vi "诊断标定3.vi"(8 "CAN端口":u16(ring), 9 "设备索引号":u16(ring), 10 "CAN卡类型":u32(ring)=21) -> ()   [LabVIEW 2013] (continued)
                          n3577 = local write "1 7"(TRUE ("1 7")) -> ()
                        }
                        frame 2 {
                          n3578 = local write "1 8"(TRUE ("1 8")) -> ()
                        }
                        frame 3 {
                          n3579 = local write "1 9"(TRUE ("1 9")) -> ()
                        }
                        frame 5 {
                          n3580 = local write "1 10"(TRUE ("1 10")) -> ()
                        }
                        frame 4 {
                          n3581 = local write "1 12"(TRUE ("1 10")) -> ()
                        }
                      }
                      n3582 = local write "等级 2"(w5186) -> ()
                    }
                  }
                  n3583 = Array Size(array=w4905) -> (size(s)=w4904:i32)
                  n3584 = local write "命令"(w4906) -> ()
                  n3585 = Build Array(w4909) -> (w4908:u8[])
                  n3586 = while {
                    tunnel: w4906 -> [w4943]
                    tunnel: w4910 -> [w4942]
                    tunnel: w4908 -> [w4941]
                    tunnel: w4904 -> [w4937]
                    tunnel: w4901 -> [w4940]
                    tunnel: w4899 -> [w4934]
                    tunnel: [w4933] -> w4898
                    shift-right: [w4932] -> _
                    shift-left: w4907 -> [w4913]
                    shift-right: [w4923] -> _
                    shift-left: w4905 -> [w4912]
                    i -> [w4938]
                    stop <- w4933 stop-if-true
                    n3587 = local read "强制终止读写标记"() -> (w4929:bool)
                    n3588 = Array Size(array=w4913) -> (size(s)=w4931:i32)
                    n3589 = Increment(x=w4938) -> (x+1=w4939:i32)
                    n3590 = Greater Than 0?(x=w4931) -> (x > 0?=w4930:bool)
                    n3591 = Equal?(x=w4937, y=w4939) -> (x = y?=w4935:bool)
                    n3592 = Not(x=w4929) -> (.not. x?=w4928:bool)
                    n3593 = And(x=w4928, y=w4930) -> (x .and. y?=w4927:bool)
                    n3594 = Delete From Array(array=w4913, length=1 ("长度"), index=0 ("索引")) -> (deleted portion=w4919:string[], array with subset deleted=w4924:string[])
                    n3595 = Index Array(array=w4919, index=0 ("索引")) -> (element=w4917:string)
                    n3596 = Delete From Array(array=w4912, length=1 ("长度"), index=0 ("索引")) -> (deleted portion=w4915:u8[], array with subset deleted=w4920:u8[])
                    n3597 = Index Array(array=w4915, index=0 ("索引")) -> (element=w4914:u8)
                    n3598 = case shown="真" w4927 {
                      tunnel: w4943 -> [_ w4959]
                      tunnel: w4914 -> [_ w4958]
                      tunnel: w4942 -> [_ w4957]
                      tunnel: w4941 -> [_ w4956]
                      tunnel: w4917 -> [_ w4955]
                      tunnel: w4940 -> [_ w4954]
                      tunnel: w4935 -> [_ w4953]
                      tunnel: w4934 -> [_ w4952]
                      tunnel: [string[] [] w4948] -> w4932
                      tunnel: w4924 -> [_ w4951]
                      tunnel: [u8[] [] w4946] -> w4923
                      tunnel: w4920 -> [_ w4950]
                      tunnel: w4913 -> [_ w4949]
                      tunnel: w4912 -> [_ w4947]
                      frame False {
                      }
                      frame True {
                        n3599 = while {
                          tunnel: w4959 -> [w4975]
                          tunnel: w4958 -> [w4974]
                          tunnel: w4957 -> [w4973]
                          tunnel: w4956 -> [w4972]
                          tunnel: w4955 -> [w4970]
                          tunnel: w4954 -> [w4969]
                          tunnel: w4953 -> [w4968]
                          tunnel: w4952 -> [w4967]
                          tunnel: w4951 -> [w4963]
                          tunnel: w4950 -> [w4961]
                          tunnel: w4949 -> [w4964]
                          tunnel: [w4965] -> w4948
                          tunnel: w4947 -> [w4962]
                          tunnel: [w4960] -> w4946
                          i -> [w4966]
                          stop <- w4971 stop-if-true
                          n3600 = stacked-sequence {
                            seq-local: [_ _ _ _ w5122 _ _] -> [_ _ _ _ _ w5138 _]
                            tunnel: w4975 -> [_ _ _ w5114 _ _ _]
                            tunnel: w4974 -> [_ _ _ w5113 _ _ _]
                            tunnel: w4973 -> [_ _ _ w5112 _ _ _]
                            tunnel: w4972 -> [_ _ _ w5111 _ _ _]
                            tunnel: [_ _ _ _ w5123 _ _] -> w4971
                            tunnel: w4970 -> [w4977 _ _ _ _ w5137 _]
                            tunnel: w4969 -> [_ _ _ _ _ _ w5165]
                            tunnel: w4968 -> [_ _ _ _ _ _ w5163]
                            tunnel: w4967 -> [w4976 _ _ _ _ _ _]
                            tunnel: w4966 -> [_ _ _ _ _ _ _]
                            tunnel: [_ _ _ _ _ w5136 _] -> w4965
                            tunnel: w4964 -> [_ _ _ _ _ w5135 _]
                            tunnel: w4963 -> [_ _ _ _ _ w5134 _]
                            tunnel: w4962 -> [_ _ _ _ _ w5133 _]
                            tunnel: w4961 -> [_ _ _ _ _ w5132 _]
                            tunnel: [_ _ _ _ _ w5131 _] -> w4960
                            frame #0 {
                              n3601 = case shown="\"从板\"" w4976 {
                                tunnel: w4977 -> [w4978 w5069]
                                frame "主板", Default {
                                n3602 = case shown="\"电压个数\"" w4978 {
                                frame "假", Default {
                                }
                                frame "产品编号" {
                                n3603 = control-ref of="产品编号"() -> (w4980:refnum<vi>)
                                n3604 = property class="Str"(reference=w4980, "Value"="") -> ()  [unwired: 1 in, 2 out]
                                }
                                frame "电压个数" {
                                n3605 = local read "从板个数"() -> (w4981:dbl)
                                n3606 = control-ref of="项目信息"() -> (w4985:refnum<vi>)
                                n3607 = for {
                                N: w4981 -> [_]
                                tunnel: [""] -> w4984 mode=indexing
                                }
                                n3608 = call "表格数据输入-8.6.vi"("行数"=u32 0, "列数"=u32 1, "字符串数组"=w4984, "表格引用"=w4985) -> ()  [unwired: 8 in]
                                }
                                frame "通道电压数" {
                                n3609 = disable-structure shown="禁用" {
                                frame Disabled {
                                n3610 = control-ref of="项目信息"() -> (w4991:refnum<vi>)
                                n3611 = for {
                                N: 20 -> [_]
                                tunnel: [""] -> w4990 mode=indexing
                                }
                                n3612 = local read "从板个数"() -> (w4992:dbl)
                                n3613 = Increment(x=w4992) -> (x+1=w4988:dbl)
                                n3614 = call "表格数据输入-8.6.vi"("行数"=w4988, "列数"=u32 1, "字符串数组"=w4990, "表格引用"=w4991) -> ()  [unwired: 8 in]
                                }
                                frame Enabled {
                                }
                                }
                                }
                                frame "电压起始值" {
                                n3615 = disable-structure shown="禁用" {
                                frame Disabled {
                                n3616 = local read "从板个数"() -> (w4996:dbl)
                                n3617 = Increment(x=w4996) -> (x+1=w4995:dbl)
                                n3618 = control-ref of="项目信息"() -> (w5002:refnum<vi>)
                                n3619 = for {
                                N: w4995 -> [_]
                                tunnel: [""] -> w5001 mode=indexing
                                }
                                n3620 = Multiply(x=u8 1, y=w4996) -> (x*y=w4998:dbl)
                                n3621 = Add(x=w4998, y=u8 21) -> (x+y=w4994:dbl)
                                n3622 = call "表格数据输入-8.6.vi"("行数"=w4994, "列数"=u32 1, "字符串数组"=w5001, "表格引用"=w5002) -> ()  [unwired: 8 in]
                                }
                                frame Enabled {
                                }
                                }
                                }
                                frame "温度个数" {
                                n3623 = local read "从板个数"() -> (w5006:dbl)
                                n3624 = Increment(x=w5006) -> (x+1=w5005:dbl)
                                n3625 = control-ref of="项目信息"() -> (w5012:refnum<vi>)
                                n3626 = for {
                                N: w5005 -> [_]
                                tunnel: [""] -> w5011 mode=indexing
                                }
                                n3627 = Multiply(x=u8 2, y=w5006) -> (x*y=w5008:dbl)
                                n3628 = Add(x=w5008, y=u8 22) -> (x+y=w5004:dbl)
                                n3629 = call "表格数据输入-8.6.vi"("行数"=w5004, "列数"=u32 1, "字符串数组"=w5011, "表格引用"=w5012) -> ()  [unwired: 8 in]
                                }
                                frame "温度起始值" {
                                n3630 = disable-structure shown="禁用" {
                                frame Disabled {
                                n3631 = local read "从板个数"() -> (w5016:dbl)
                                n3632 = Increment(x=w5016) -> (x+1=w5015:dbl)
                                n3633 = control-ref of="项目信息"() -> (w5022:refnum<vi>)
                                n3634 = for {
                                N: w5015 -> [_]
                                tunnel: [""] -> w5021 mode=indexing
                                }
                                n3635 = Multiply(x=u8 3, y=w5016) -> (x*y=w5018:dbl)
                                n3636 = Add(x=w5018, y=u8 23) -> (x+y=w5014:dbl)
                                n3637 = call "表格数据输入-8.6.vi"("行数"=w5014, "列数"=u32 1, "字符串数组"=w5021, "表格引用"=w5022) -> ()  [unwired: 8 in]
                                }
                                frame Enabled {
                                }
                                }
                                }
                                frame "保险位置" {
                                n3638 = local read "从板个数"() -> (w5026:dbl)
                                n3639 = control-ref of="项目信息"() -> (w5032:refnum<vi>)
                                n3640 = for {
                                N: 10 -> [_]
                                tunnel: [""] -> w5031 mode=indexing
                                }
                                n3641 = Multiply(x=u8 4, y=w5026) -> (x*y=w5028:dbl)
                                n3642 = Add(x=w5028, y=u8 24) -> (x+y=w5025:dbl)
                                n3643 = call "表格数据输入-8.6.vi"("行数"=w5025, "列数"=u32 1, "字符串数组"=w5031, "表格引用"=w5032) -> ()  [unwired: 8 in]
                                }
                                frame "电池额定实际容量" {
                                w5034 = 0.0 ("值")
                                n3644 = control-ref of="电池实际容量(A)"() -> (w5035:refnum<vi>)
                                n3645 = control-ref of="电池额定容量(A)"() -> (w5036:refnum<vi>)
                                n3646 = property class="DigNum (严格)"(reference=w5035, "Value"=w5034) -> ()  [unwired: 1 in, 2 out]
                                n3647 = property class="DigNum (严格)"(reference=w5036, "Value"=w5034) -> ()  [unwired: 1 in, 2 out]
                                }
                                frame "SOC" {
                                n3648 = control-ref of="SOC(%)"() -> (w5037:refnum<vi>)
                                n3649 = property class="DigNum (严格)"(reference=w5037, "Value"=0.0 ("值")) -> ()  [unwired: 1 in, 2 out]
                                }
                                frame "配置文件版本" {
                                n3650 = control-ref of="配置文件版本"() -> (w5039:refnum<vi>)
                                n3651 = property class="Str"(reference=w5039, "Value"="" ("值")) -> ()  [unwired: 1 in, 2 out]
                                }
                                frame "参数修改记录" {
                                n3652 = control-ref of="使用者"() -> (w5042:refnum<vi>)
                                n3653 = control-ref of="系统时钟"() -> (w5043:refnum<vi>)
                                n3654 = property class="DigNum (严格)"(reference=w5042, "Value"=0.0 ("值")) -> ()  [unwired: 1 in, 2 out]
                                n3655 = property class="Str"(reference=w5043, "Value"="" ("值")) -> ()  [unwired: 1 in, 2 out]
                                }
                                frame "校正时钟" {
                                n3656 = control-ref of="系统时钟"() -> (w5045:refnum<vi>)
                                n3657 = property class="Str"(reference=w5045, "Value"="" ("值")) -> ()  [unwired: 1 in, 2 out]
                                }
                                frame "车牌号" {
                                n3658 = control-ref of="车架(牌)号"() -> (w5047:refnum<vi>)
                                n3659 = property class="Str"(reference=w5047, "Value"="" ("值")) -> ()  [unwired: 1 in, 2 out]
                                }
                                frame "SOH" {
                                n3660 = control-ref of="SOH(%)"() -> (w5050:refnum<vi>)
                                n3661 = property class="DigNum (严格)"(reference=w5050, "Value"=0.0 ("值")) -> ()  [unwired: 1 in, 2 out]
                                }
                                frame "一级故障阀值" {
                                n3662 = local write "一级故障"(T10 {"总电压过高"=0.0, "整组电压不均衡"=0.0, "SOC过高"=0.0, "单体电压过高"=0.0, "总电压过低"=0.0, "温度过高"=0.0, "温度过低"=0.0, "单组电压不均衡"=0.0, "整组温度不均衡"=0.0, "单组温度不均衡"=0.0, "单体电压过低"=0.0, "充电电流过高"=0.0, "放电电流过高"=0.0, "SOC过低"=0.0, "内阻过大"=0.0, "极柱温度过高"=0.0, "SOH过低"=0.0} ("一级故障")) -> ()
                                }
                                frame "二级故障阀值" {
                                n3663 = local write "一级故障 2"(T10 {"总电压过高"=0.0, "整组电压不均衡"=0.0, "SOC过高"=0.0, "单体电压过高"=0.0, "总电压过低"=0.0, "温度过高"=0.0, "温度过低"=0.0, "单组电压不均衡"=0.0, "整组温度不均衡"=0.0, "单组温度不均衡"=0.0, "单体电压过低"=0.0, "充电电流过高"=0.0, "放电电流过高"=0.0, "SOC过低"=0.0, "内阻过大"=0.0, "极柱温度过高"=0.0, "SOH过低"=0.0} ("一级故障")) -> ()
                                }
                                frame "三级故障阀值" {
                                n3664 = local write "一级故障 3"(T10 {"总电压过高"=0.0, "整组电压不均衡"=0.0, "SOC过高"=0.0, "单体电压过高"=0.0, "总电压过低"=0.0, "温度过高"=0.0, "温度过低"=0.0, "单组电压不均衡"=0.0, "整组温度不均衡"=0.0, "单组温度不均衡"=0.0, "单体电压过低"=0.0, "充电电流过高"=0.0, "放电电流过高"=0.0, "SOC过低"=0.0, "内阻过大"=0.0, "极柱温度过高"=0.0, "SOH过低"=0.0} ("一级故障")) -> ()
                                }
                                frame "加热控制参数" {
                                n3665 = local write "加热控制参数"(T11 {"风机开启温度"=0.0, "风机关闭温度"=0.0, "加热开启温度"=0.0, "加热关闭温度"=0.0, "风机开启温差"=0.0, "风机关闭温差"=0.0, "加热关闭温差"=0.0} ("加热控制参数")) -> ()
                                }
                                frame "充电控制参数" {
                                n3666 = local write "一级故障 5"(T12 {"最大允许单体电压"=0.0, "最大允许总电压"=0.0, "最小允许单体电压"=0.0, "最大允许充电电流"=0.0, "最小允许充电电流"=0.0, "最大允许充电温度"=0.0, "最小允许充电温度"=0.0, "电流步长"=0.0} ("一级故障 5")) -> ()
                                }
                                frame "电池信息1" {
                                w5056 = ""
                                w5057 = 0.0 ("电池串联")
                                n3667 = local read "电池信息"() -> (w5059:T13)
                                n3668 = Bundle By Name(cluster=w5059, "电池串联"=w5057, "电池并联"=w5057, "电池包额定容量"=w5057, "电池包额定能量(kWh)"=w5057, "电池包额定总电压"=w5057, "实际容量"=w5057, "电池厂家"=w5056, "电池类型"=w5056, "电池生产日期"=w5056) -> (w5058:T13)
                                n3669 = local write "电池信息"(w5058) -> ()
                                }
                                frame "电池包组号" {
                                n3670 = local read "电池信息"() -> (w5062:T13)
                                n3671 = Bundle By Name(cluster=w5062, "电池包组号"="") -> (w5061:T13)
                                n3672 = local write "电池信息"(w5061) -> ()
                                }
                                frame "充放电安时" {
                                w5063 = 0.0 ("累计充电总安时")
                                n3673 = local read "电池信息"() -> (w5065:T13)
                                n3674 = Bundle By Name(cluster=w5065, "累计充电总安时"=w5063, "累计放电总安时"=w5063) -> (w5064:T13)
                                n3675 = local write "电池信息"(w5064) -> ()
                                }
                                frame "电池充放电次数" {
                                w5066 = 0.0 ("累计充电总安时")
                                n3676 = local read "电池信息"() -> (w5068:T13)
                                n3677 = Bundle By Name(cluster=w5068, "电池充满次数"=w5066, "电池放空次数"=w5066, "电池充电次数"=w5066) -> (w5067:T13)
                                n3678 = local write "电池信息"(w5067) -> ()
                                }
                                }
                                }
                                frame "从板" {
                                n3679 = case shown="\"电压起始值\"" w5069 {
                                frame "假", Default {
                                }
                                frame "电压起始值" {
                                n3680 = control-ref of="项目信息 2"() -> (w5070:refnum<vi>)
                                n3681 = for {
                                N: 1 -> [_]
                                tunnel: [""] -> w5074 mode=indexing
                                }
                                n3682 = call "表格数据输入-8.6.vi"("行数"=u32 0, "列数"=u32 1, "字符串数组"=w5074, "表格引用"=w5070) -> ()  [unwired: 8 in]
                                }
                                frame "通道电压个数" {
                                n3683 = control-ref of="项目信息 2"() -> (w5076:refnum<vi>)
                                n3684 = for {
                                N: 5 -> [_]
                                tunnel: [""] -> w5080 mode=indexing
                                }
                                n3685 = call "表格数据输入-8.6.vi"("行数"=u32 22, "列数"=u32 1, "字符串数组"=w5080, "表格引用"=w5076) -> ()  [unwired: 8 in]
                                }
                                frame "保险位置" {
                                n3686 = control-ref of="项目信息 2"() -> (w5082:refnum<vi>)
                                n3687 = for {
                                N: 10 -> [_]
                                tunnel: [""] -> w5086 mode=indexing
                                }
                                n3688 = call "表格数据输入-8.6.vi"("行数"=u32 2, "列数"=u32 1, "字符串数组"=w5086, "表格引用"=w5082) -> ()  [unwired: 8 in]
                                }
                                frame "温度起始值" {
                                n3689 = control-ref of="项目信息 2"() -> (w5088:refnum<vi>)
                                n3690 = for {
                                N: 1 -> [_]
                                tunnel: [""] -> w5092 mode=indexing
                                }
                                n3691 = call "表格数据输入-8.6.vi"("行数"=u32 1, "列数"=u32 1, "字符串数组"=w5092, "表格引用"=w5088) -> ()  [unwired: 8 in]
                                }
                                frame "加热控制参数" {
                                n3692 = local write "加热控制参数"(T11 {"风机开启温度"=0.0, "风机关闭温度"=0.0, "加热开启温度"=0.0, "加热关闭温度"=0.0, "风机开启温差"=0.0, "风机关闭温差"=0.0, "加热关闭温差"=0.0} ("加热控制参数")) -> ()
                                }
                                frame "一级故障阀值" {
                                n3693 = local write "一级故障 6"(T15 {"电压过高"=0.0, "电压过低"=0.0, "温度过高"=0.0, "温度过低"=0.0, "电压不均衡(V)"=0.0, "温度不均衡"=0.0, "SOC过低"=0.0} ("一级故障 6")) -> ()
                                }
                                frame "二级故障阀值" {
                                n3694 = local write "一级故障 7"(T15 {"电压过高"=0.0, "电压过低"=0.0, "温度过高"=0.0, "温度过低"=0.0, "电压不均衡(V)"=0.0, "温度不均衡"=0.0, "SOC过低"=0.0} ("一级故障 7")) -> ()
                                }
                                frame "三级故障阀值" {
                                n3695 = local write "一级故障 8"(T15 {"电压过高"=0.0, "电压过低"=0.0, "温度过高"=0.0, "温度过低"=0.0, "电压不均衡(V)"=0.0, "温度不均衡"=0.0, "SOC过低"=0.0} ("一级故障 7")) -> ()
                                }
                                frame "均衡参数" {
                                n3696 = local write "均衡参数"(T17 {"充电结束电压(90%)"=0.0, "充电结束电压(91%)"=0.0, "充电结束电压(92%)"=0.0, "充电结束电压(93%)"=0.0, "充电结束电压(94%)"=0.0, "均衡计算-电压高阀值1级"=0.0, "均衡计算-电压高阀值2级"=0.0, "均衡计算-电压低阀值1级"=0.0, "均衡计算-电压低阀值2级"=0.0, "均衡计算-最低电压阀值"=0.0, "均衡停止-最低电压阀值"=0.0, "均衡计算-电压极差阀值"=0.0, "充电结束电压(95%)"=0.0, "充电结束电压(96%)"=0.0, "充电结束电压(97%)"=0.0, "充电结束电压(98%)"=0.0, "充电结束电压(99%)"=0.0, "充电结束电压(100%)"=0.0} ("均衡参数")) -> ()
                                }
                                frame "均衡阀值" {
                                w5099 = sgl 0.0 ("均衡计算-电压高阀值1级")
                                n3697 = local read "均衡参数"() -> (w5100:T17)
                                n3698 = Bundle By Name(cluster=w5100, "均衡计算-电压高阀值1级"=w5099, "均衡计算-电压高阀值2级"=w5099, "均衡计算-电压低阀值1级"=w5099, "均衡计算-电压低阀值2级"=w5099, "均衡计算-最低电压阀值"=w5099, "均衡停止-最低电压阀值"=w5099, "均衡计算-电压极差阀值"=w5099) -> (w5101:T17)
                                n3699 = local write "均衡参数"(w5101) -> ()
                                }
                                frame "充电结束电压" {
                                w5102 = sgl 0.0 ("均衡计算-电压高阀值1级")
                                n3700 = local read "均衡参数"() -> (w5103:T17)
                                n3701 = Bundle By Name(cluster=w5103, "充电结束电压(90%)"=w5102, "充电结束电压(91%)"=w5102, "充电结束电压(92%)"=w5102, "充电结束电压(93%)"=w5102, "充电结束电压(94%)"=w5102, "充电结束电压(95%)"=w5102, "充电结束电压(96%)"=w5102, "充电结束电压(97%)"=w5102, "充电结束电压(98%)"=w5102, "充电结束电压(99%)"=w5102, "充电结束电压(100%)"=w5102) -> (w5104:T17)
                                n3702 = local write "均衡参数"(w5104) -> ()
                                }
                                }
                                }
                              }
                            }
                            frame #1 {
                              w5105 = FALSE ("流控帧")
                              w5106 = TRUE ("流控帧 2")
                              n3703 = global write "EV05全局变量1.vi" "写入超时"(w5105) -> ()
                              n3704 = global write "EV05全局变量1.vi" "流控帧"(w5105) -> ()
                              n3705 = local write "写?"(w5105) -> ()
                              n3706 = local write "消除"(w5106) -> ()
                              n3707 = local write "控制1"(w5106) -> ()
                              n3708 = global write "EV05全局变量1.vi" "流控帧 2"(w5106) -> ()
                            }
                            frame #2 {
                              n3709 = Wait Until Next ms Multiple(millisecond multiple=u32 300 ("毫秒倍数")) -> ()  [unwired: 1 out]
                            }
                            frame #3 {
                              n3710 = local read "设备索引号"() -> (w5109:u16)
                              n3711 = local read "CAN卡类型"() -> (w5110:u32)
                              n3712 = local read "CAN端口"() -> (w5108:u16)
                              n3713 = local write "命令序号"(w5113) -> ()
                              n3714 = stacked-sequence {
                                tunnel: w5114 -> [_ w5121]
                                tunnel: w5113 -> [_ w5120]
                                tunnel: w5112 -> [_ w5119]
                                tunnel: w5111 -> [_ w5118]
                                tunnel: w5110 -> [_ w5117]
                                tunnel: w5109 -> [_ w5116]
                                tunnel: w5108 -> [_ w5115]
                                frame #0 {
                                }
                                frame #1 {
                                n3715 = call "多帧发送机制(EV05).vi"("can卡类型"=w5117, "设备索引号"=w5116, "CAN端口"=w5115, "命令"=w5121, "板号"=w5119, "命令序号"=w5120, "输入数据"=w5118) -> ()  [unwired: 1 in, 12 out]
                                }
                              }
                            }
                            frame #4 {
                              n3716 = while {
                                tunnel: [w5126] -> w5123
                                tunnel: [w5125] -> w5122
                                i -> [w5129]
                                stop <- w5126 stop-if-true
                                n3717 = local read "强制终止读写标记"() -> (w5124:bool)
                                n3718 = global read "EV05全局变量1.vi" "写入超时"() -> (w5125:bool)
                                n3719 = Greater Or Equal?(x=w5129, y=20) -> (x >= y?=w5127:bool)
                                n3720 = Compound Arithmetic op=OR(w5124, w5125, w5127) -> (w5126:bool)
                                n3721 = Wait Until Next ms Multiple(millisecond multiple=u32 100 ("毫秒倍数")) -> ()  [unwired: 1 out]
                              }
                            }
                            frame #5 {
                              n3722 = case shown="假" w5138 {
                                tunnel: w5137 -> [w5149 _]
                                tunnel: [w5144 w5161] -> w5136
                                tunnel: w5135 -> [w5143 _]
                                tunnel: w5134 -> [w5142 w5161]
                                tunnel: [w5141 w5160] -> w5131
                                tunnel: w5133 -> [w5140 _]
                                tunnel: w5132 -> [w5139 w5160]
                                frame False {
                                n3723 = local read "重试次数"() -> (w5148:u8)
                                n3724 = Increment(x=w5148) -> (x+1=w5147:u8)
                                n3725 = local write "重试次数"(w5147) -> ()
                                n3726 = Greater Or Equal?(x=w5147, y=u8 4) -> (x >= y?=w5146:bool)
                                n3727 = case shown="真" w5146 {
                                tunnel: w5149 -> [_ w5154]
                                tunnel: [w5151 w5153] -> w5144
                                tunnel: w5143 -> [w5151 _]
                                tunnel: w5142 -> [_ w5153]
                                tunnel: [w5150 w5152] -> w5141
                                tunnel: w5140 -> [w5150 _]
                                tunnel: w5139 -> [_ w5152]
                                frame False {
                                }
                                frame True {
                                n3728 = control-ref of="结果"() -> (w5156:refnum<vi>)
                                n3729 = Concatenate Strings(w5154, "     读取失败" ("字符串")) -> (w5158:string)
                                n3730 = Build Array(w5158) -> (w5155:string[])
                                n3731 = call "表格编辑.vi"("新元素/子数组"=w5155, "活动单元格:单元格背景色"=u32 16740749, "MCListbox引用句柄"=w5156) -> ()  [unwired: 9 out]
                                }
                                }
                                }
                                frame True {
                                }
                              }
                            }
                            frame #6 {
                              n3732 = And(x=w5163, y=w5165) -> (x .and. y?=w5164:bool)
                              n3733 = case shown="真" w5164 {
                                frame False {
                                }
                                frame True {
                                n3734 = local write "强制终止读写标记"(FALSE ("强制停止")) -> ()
                                n3735 = control-ref of="结果"() -> (w5168:refnum<vi>)
                                n3736 = Concatenate Strings("读取完成" ("字符串")) -> (w5170:string)
                                n3737 = Build Array(w5170) -> (w5167:string[])
                                n3738 = call "表格编辑.vi"("新元素/子数组"=w5167, "活动单元格:单元格背景色"=u32 21937, "MCListbox引用句柄"=w5168) -> ()  [unwired: 9 out]
                                }
                              }
                              n3739 = Wait (ms)(milliseconds to wait=u32 100 ("等待时间（毫秒）")) -> ()  [unwired: 1 out]
                            }
                          }
                        }
                      }
                    }
                    n3740 = local read "强制终止读写标记"() -> (w4936:bool)
                    n3741 = Or(x=w4936, y=w4935) -> (x .or. y?=w4933:bool)
                  }
                }
              }
              frame #2 {
                n3742 = case shown="假" w5261 {
                  tunnel: w5262 -> [w5263 _]
                  frame False {
                    n3743 = case shown="\"主板\", 默认" w5263 {
                      frame "主板", Default {
                        n3744 = global read "读配置文件全局.vi" "电池额定实际容量判定"() -> (w5277:bool)
                        n3745 = global read "读配置文件全局.vi" "电池充放电次数判定"() -> (w5266:bool)
                        n3746 = global read "读配置文件全局.vi" "加热控制参数判定"() -> (w5264:bool)
                        n3747 = global read "读配置文件全局.vi" "配置文件版本判定"() -> (w5276:bool)
                        n3748 = global read "读配置文件全局.vi" "充电控制参数判定"() -> (w5270:bool)
                        n3749 = global read "读配置文件全局.vi" "通道电压数判定"() -> (w5282:bool)
                        n3750 = global read "读配置文件全局.vi" "电压起始值判定"() -> (w5281:bool)
                        n3751 = global read "读配置文件全局.vi" "温度起始值判定"() -> (w5279:bool)
                        n3752 = global read "读配置文件全局.vi" "充放电安时判定"() -> (w5268:bool)
                        n3753 = global read "读配置文件全局.vi" "电池包组号判定"() -> (w5267:bool)
                        n3754 = global read "读配置文件全局.vi" "电池信息1判定"() -> (w5269:bool)
                        n3755 = global read "读配置文件全局.vi" "从板个数判定"() -> (w5285:bool)
                        n3756 = global read "读配置文件全局.vi" "产品编号判定"() -> (w5284:bool)
                        n3757 = global read "读配置文件全局.vi" "电压个数判定"() -> (w5283:bool)
                        n3758 = global read "读配置文件全局.vi" "温度个数判定"() -> (w5280:bool)
                        n3759 = global read "读配置文件全局.vi" "保险位置判定"() -> (w5278:bool)
                        n3760 = global read "读配置文件全局.vi" "一级故障判定"() -> (w5273:bool)
                        n3761 = global read "读配置文件全局.vi" "二级故障判定"() -> (w5272:bool)
                        n3762 = global read "读配置文件全局.vi" "三级故障判定"() -> (w5271:bool)
                        n3763 = global read "读配置文件全局.vi" "车牌号判定"() -> (w5275:bool)
                        n3764 = global read "读配置文件全局.vi" "SOH判定"() -> (w5274:bool)
                        n3765 = Build Array(w5285, w5284, w5283, w5282, w5281, w5280, w5279, w5278, w5277, w5276, w5275, w5274, w5273, w5272, w5271, w5270, w5269, w5268, w5267, w5266, w5264) -> (w5265:bool[])
                        n3766 = And Array Elements(Boolean array=w5265) -> (logical AND=w5286:bool)
                        n3767 = disable-structure shown="禁用" {
                          frame Disabled {
                            n3768 = global read "读配置文件全局.vi" "SOC判定"() -> ()  [unwired: 1 out]
                          }
                          frame Enabled {
                          }
                        }
                        n3769 = case shown="假" w5286 {
                          tunnel: w5265 -> [_ w5291]
                          frame True {
                            n3770 = control-ref of="结果"() -> (w5289:refnum<vi>)
                            n3771 = Build Array("全部判定成功!!!!!!!!") -> (w5290:string[])
                            n3772 = call "表格编辑.vi"("新元素/子数组"=w5290, "活动单元格:单元格背景色"=u32 6618880, "MCListbox引用句柄"=w5289) -> ()  [unwired: 9 out]
                          }
                          frame False {
                            n3773 = stacked-sequence {
                              tunnel: w5291 -> [_ w5296]
                              frame #0 {
                                n3774 = control-ref of="结果"() -> (w5294:refnum<vi>)
                                n3775 = Build Array("全部判定失败!!!!!") -> (w5295:string[])
                                n3776 = call "表格编辑.vi"("新元素/子数组"=w5295, "活动单元格:单元格背景色"=u32 16711680, "MCListbox引用句柄"=w5294) -> ()  [unwired: 9 out]
                              }
                              frame #1 {
                                n3777 = for {
                                tunnel: w5296 -> [w5298] mode=indexing
                                i -> [w5297]
                                n3778 = case shown="20" w5297 {
                                tunnel: w5298 -> [w5299 w5304 w5309 w5314 w5319 w5324 w5329 w5334 w5339 w5344 w5349 w5354 w5359 w5364 w5369 w5374 w5379 w5384 w5389 w5394 w5399 _]
                                frame 0 {
                                n3779 = case shown="假" w5299 {
                                frame False {
                                n3780 = control-ref of="结果"() -> (w5302:refnum<vi>)
                                n3781 = Build Array("从板个数判定失败!") -> (w5303:string[])
                                n3782 = call "表格编辑.vi"("新元素/子数组"=w5303, "活动单元格:单元格背景色"=u32 16711680, "MCListbox引用句柄"=w5302) -> ()  [unwired: 9 out]
                                }
                                frame True {
                                }
                                }
                                }
                                frame 1 {
                                n3783 = case shown="假" w5304 {
                                frame False {
                                n3784 = control-ref of="结果"() -> (w5307:refnum<vi>)
                                n3785 = Build Array("产品编号判定失败!") -> (w5308:string[])
                                n3786 = call "表格编辑.vi"("新元素/子数组"=w5308, "活动单元格:单元格背景色"=u32 16711680, "MCListbox引用句柄"=w5307) -> ()  [unwired: 9 out]
                                }
                                frame True {
                                }
                                }
                                }
                                frame 2 {
                                n3787 = case shown="假" w5309 {
                                frame False {
                                n3788 = control-ref of="结果"() -> (w5312:refnum<vi>)
                                n3789 = Build Array("电压个数判定失败!") -> (w5313:string[])
                                n3790 = call "表格编辑.vi"("新元素/子数组"=w5313, "活动单元格:单元格背景色"=u32 16711680, "MCListbox引用句柄"=w5312) -> ()  [unwired: 9 out]
                                }
                                frame True {
                                }
                                }
                                }
                                frame 3 {
                                n3791 = case shown="假" w5314 {
                                frame False {
                                n3792 = control-ref of="结果"() -> (w5317:refnum<vi>)
                                n3793 = Build Array("通道电压数判定失败!") -> (w5318:string[])
                                n3794 = call "表格编辑.vi"("新元素/子数组"=w5318, "活动单元格:单元格背景色"=u32 16711680, "MCListbox引用句柄"=w5317) -> ()  [unwired: 9 out]
                                }
                                frame True {
                                }
                                }
                                }
                                frame 4 {
                                n3795 = case shown="假" w5319 {
                                frame False {
                                n3796 = control-ref of="结果"() -> (w5322:refnum<vi>)
                                n3797 = Build Array("电压起始值判定失败!") -> (w5323:string[])
                                n3798 = call "表格编辑.vi"("新元素/子数组"=w5323, "活动单元格:单元格背景色"=u32 16711680, "MCListbox引用句柄"=w5322) -> ()  [unwired: 9 out]
                                }
                                frame True {
                                }
                                }
                                }
                                frame 5 {
                                n3799 = case shown="假" w5324 {
                                frame False {
                                n3800 = control-ref of="结果"() -> (w5327:refnum<vi>)
                                n3801 = Build Array("温度个数判定失败!") -> (w5328:string[])
                                n3802 = call "表格编辑.vi"("新元素/子数组"=w5328, "活动单元格:单元格背景色"=u32 16711680, "MCListbox引用句柄"=w5327) -> ()  [unwired: 9 out]
                                }
                                frame True {
                                }
                                }
                                }
                                frame 6 {
                                n3803 = case shown="假" w5329 {
                                frame False {
                                n3804 = control-ref of="结果"() -> (w5332:refnum<vi>)
                                n3805 = Build Array("温度起始值判定失败!") -> (w5333:string[])
                                n3806 = call "表格编辑.vi"("新元素/子数组"=w5333, "活动单元格:单元格背景色"=u32 16711680, "MCListbox引用句柄"=w5332) -> ()  [unwired: 9 out]
                                }
                                frame True {
                                }
                                }
                                }
                                frame 7 {
                                n3807 = case shown="假" w5334 {
                                frame False {
                                n3808 = control-ref of="结果"() -> (w5337:refnum<vi>)
                                n3809 = Build Array("保险位置判定失败!") -> (w5338:string[])
                                n3810 = call "表格编辑.vi"("新元素/子数组"=w5338, "活动单元格:单元格背景色"=u32 16711680, "MCListbox引用句柄"=w5337) -> ()  [unwired: 9 out]
                                }
                                frame True {
                                }
                                }
                                }
                                frame 8 {
                                n3811 = case shown="假" w5339 {
                                frame False {
                                n3812 = control-ref of="结果"() -> (w5342:refnum<vi>)
                                n3813 = Build Array("电池额定实际容量判定失败!") -> (w5343:string[])
                                n3814 = call "表格编辑.vi"("新元素/子数组"=w5343, "活动单元格:单元格背景色"=u32 16711680, "MCListbox引用句柄"=w5342) -> ()  [unwired: 9 out]
                                }
                                frame True {
                                }
                                }
                                }
                                frame 9 {
                                n3815 = case shown="假" w5344 {
                                frame False {
                                n3816 = control-ref of="结果"() -> (w5347:refnum<vi>)
                                n3817 = Build Array("配置文件版本判定失败!") -> (w5348:string[])
                                n3818 = call "表格编辑.vi"("新元素/子数组"=w5348, "活动单元格:单元格背景色"=u32 16711680, "MCListbox引用句柄"=w5347) -> ()  [unwired: 9 out]
                                }
                                frame True {
                                }
                                }
                                }
                                frame 10 {
                                n3819 = case shown="假" w5349 {
                                frame False {
                                n3820 = control-ref of="结果"() -> (w5352:refnum<vi>)
                                n3821 = Build Array("车牌号判定失败!") -> (w5353:string[])
                                n3822 = call "表格编辑.vi"("新元素/子数组"=w5353, "活动单元格:单元格背景色"=u32 16711680, "MCListbox引用句柄"=w5352) -> ()  [unwired: 9 out]
                                }
                                frame True {
                                }
                                }
                                }
                                frame 11 {
                                n3823 = case shown="假" w5354 {
                                frame False {
                                n3824 = control-ref of="结果"() -> (w5357:refnum<vi>)
                                n3825 = Build Array("SOH判定失败!") -> (w5358:string[])
                                n3826 = call "表格编辑.vi"("新元素/子数组"=w5358, "活动单元格:单元格背景色"=u32 16711680, "MCListbox引用句柄"=w5357) -> ()  [unwired: 9 out]
                                }
                                frame True {
                                }
                                }
                                }
                                frame 12 {
                                n3827 = case shown="假" w5359 {
                                frame False {
                                n3828 = control-ref of="结果"() -> (w5362:refnum<vi>)
                                n3829 = Build Array("一级故障阀值判定失败!") -> (w5363:string[])
                                n3830 = call "表格编辑.vi"("新元素/子数组"=w5363, "活动单元格:单元格背景色"=u32 16711680, "MCListbox引用句柄"=w5362) -> ()  [unwired: 9 out]
                                }
                                frame True {
                                }
                                }
                                }
                                frame 13 {
                                n3831 = case shown="假" w5364 {
                                frame False {
                                n3832 = control-ref of="结果"() -> (w5367:refnum<vi>)
                                n3833 = Build Array("二级故障阀值判定失败!") -> (w5368:string[])
                                n3834 = call "表格编辑.vi"("新元素/子数组"=w5368, "活动单元格:单元格背景色"=u32 16711680, "MCListbox引用句柄"=w5367) -> ()  [unwired: 9 out]
                                }
                                frame True {
                                }
                                }
                                }
                                frame 14 {
                                n3835 = case shown="假" w5369 {
                                frame False {
                                n3836 = control-ref of="结果"() -> (w5372:refnum<vi>)
                                n3837 = Build Array("三级故障阀值判定失败!") -> (w5373:string[])
                                n3838 = call "表格编辑.vi"("新元素/子数组"=w5373, "活动单元格:单元格背景色"=u32 16711680, "MCListbox引用句柄"=w5372) -> ()  [unwired: 9 out]
                                }
                                frame True {
                                }
                                }
                                }
                                frame 15 {
                                n3839 = case shown="假" w5374 {
                                frame False {
                                n3840 = control-ref of="结果"() -> (w5377:refnum<vi>)
                                n3841 = Build Array("充电控制参数判定失败!") -> (w5378:string[])
                                n3842 = call "表格编辑.vi"("新元素/子数组"=w5378, "活动单元格:单元格背景色"=u32 16711680, "MCListbox引用句柄"=w5377) -> ()  [unwired: 9 out]
                                }
                                frame True {
                                }
                                }
                                }
                                frame 16 {
                                n3843 = case shown="假" w5379 {
                                frame False {
                                n3844 = control-ref of="结果"() -> (w5382:refnum<vi>)
                                n3845 = Build Array("电池信息1判定失败!") -> (w5383:string[])
                                n3846 = call "表格编辑.vi"("新元素/子数组"=w5383, "活动单元格:单元格背景色"=u32 16711680, "MCListbox引用句柄"=w5382) -> ()  [unwired: 9 out]
                                }
                                frame True {
                                }
                                }
                                }
                                frame 17 {
                                n3847 = case shown="假" w5384 {
                                frame False {
                                n3848 = control-ref of="结果"() -> (w5387:refnum<vi>)
                                n3849 = Build Array("充放电安时判定失败!") -> (w5388:string[])
                                n3850 = call "表格编辑.vi"("新元素/子数组"=w5388, "活动单元格:单元格背景色"=u32 16711680, "MCListbox引用句柄"=w5387) -> ()  [unwired: 9 out]
                                }
                                frame True {
                                }
                                }
                                }
                                frame 18 {
                                n3851 = case shown="假" w5389 {
                                frame False {
                                n3852 = control-ref of="结果"() -> (w5392:refnum<vi>)
                                n3853 = Build Array("电池包组号判定失败!") -> (w5393:string[])
                                n3854 = call "表格编辑.vi"("新元素/子数组"=w5393, "活动单元格:单元格背景色"=u32 16711680, "MCListbox引用句柄"=w5392) -> ()  [unwired: 9 out]
                                }
                                frame True {
                                }
                                }
                                }
                                frame 19 {
                                n3855 = case shown="假" w5394 {
                                frame False {
                                n3856 = control-ref of="结果"() -> (w5397:refnum<vi>)
                                n3857 = Build Array("电池充放电次数判定失败!") -> (w5398:string[])
                                n3858 = call "表格编辑.vi"("新元素/子数组"=w5398, "活动单元格:单元格背景色"=u32 16711680, "MCListbox引用句柄"=w5397) -> ()  [unwired: 9 out]
                                }
                                frame True {
                                }
                                }
                                }
                                frame 20 {
                                n3859 = case shown="假" w5399 {
                                frame False {
                                n3860 = control-ref of="结果"() -> (w5402:refnum<vi>)
                                n3861 = Build Array("加热控制参数判定失败!") -> (w5403:string[])
                                n3862 = call "表格编辑.vi"("新元素/子数组"=w5403, "活动单元格:单元格背景色"=u32 16711680, "MCListbox引用句柄"=w5402) -> ()  [unwired: 9 out]
                                }
                                frame True {
                                }
                                }
                                }
                                frame 99, Default {
                                }
                                }
                                }
                              }
                            }
                          }
                        }
                      }
                      frame "从板" {
                        n3863 = global read "读配置文件全局2.vi" "电压起始值判定"() -> (w5412:bool)
                        n3864 = global read "读配置文件全局2.vi" "温度起始值判定"() -> (w5409:bool)
                        n3865 = global read "读配置文件全局2.vi" "加热控制参数判定"() -> (w5404:bool)
                        n3866 = global read "读配置文件全局2.vi" "通道电压判定"() -> (w5411:bool)
                        n3867 = global read "读配置文件全局2.vi" "保险位置判定"() -> (w5410:bool)
                        n3868 = global read "读配置文件全局2.vi" "一级故障判定"() -> (w5407:bool)
                        n3869 = global read "读配置文件全局2.vi" "二级故障判定"() -> (w5406:bool)
                        n3870 = global read "读配置文件全局2.vi" "三级故障判定"() -> (w5405:bool)
                        n3871 = global read "读配置文件全局2.vi" "从板号判定"() -> (w5413:bool)
                        n3872 = Build Array(w5413, w5412, w5411, w5410, w5409, w5407, w5406, w5405, w5404) -> (w5408:bool[])
                        n3873 = And Array Elements(Boolean array=w5408) -> (logical AND=w5414:bool)
                        n3874 = case shown="假" w5414 {
                          tunnel: w5408 -> [_ w5419]
                          frame True {
                            n3875 = control-ref of="结果"() -> (w5417:refnum<vi>)
                            n3876 = Build Array("读取判定成功!!!!!!!!") -> (w5418:string[])
                            n3877 = call "表格编辑.vi"("新元素/子数组"=w5418, "活动单元格:单元格背景色"=u32 6618880, "MCListbox引用句柄"=w5417) -> ()  [unwired: 9 out]
                          }
                          frame False {
                            n3878 = stacked-sequence {
                              tunnel: w5419 -> [_ w5424]
                              frame #0 {
                                n3879 = control-ref of="结果"() -> (w5422:refnum<vi>)
                                n3880 = Build Array("读取判定失败!!!!!") -> (w5423:string[])
                                n3881 = call "表格编辑.vi"("新元素/子数组"=w5423, "活动单元格:单元格背景色"=u32 16711680, "MCListbox引用句柄"=w5422) -> ()  [unwired: 9 out]
                              }
                              frame #1 {
                                n3882 = for {
                                tunnel: w5424 -> [w5425] mode=indexing
                                i -> [w5426]
                                n3883 = case shown="0" w5426 {
                                tunnel: w5425 -> [w5427 w5432 w5437 w5442 w5447 w5452 w5457 w5462 w5467 _]
                                frame 0 {
                                n3884 = case shown="假" w5427 {
                                frame False {
                                n3885 = control-ref of="结果"() -> (w5430:refnum<vi>)
                                n3886 = Build Array("从板号判定失败!") -> (w5431:string[])
                                n3887 = call "表格编辑.vi"("新元素/子数组"=w5431, "活动单元格:单元格背景色"=u32 16711680, "MCListbox引用句柄"=w5430) -> ()  [unwired: 9 out]
                                }
                                frame True {
                                }
                                }
                                }
                                frame 1 {
                                n3888 = case shown="假" w5432 {
                                frame False {
                                n3889 = control-ref of="结果"() -> (w5435:refnum<vi>)
                                n3890 = Build Array("电压起始值判定失败!") -> (w5436:string[])
                                n3891 = call "表格编辑.vi"("新元素/子数组"=w5436, "活动单元格:单元格背景色"=u32 16711680, "MCListbox引用句柄"=w5435) -> ()  [unwired: 9 out]
                                }
                                frame True {
                                }
                                }
                                }
                                frame 2 {
                                n3892 = case shown="假" w5437 {
                                frame False {
                                n3893 = control-ref of="结果"() -> (w5440:refnum<vi>)
                                n3894 = Build Array("通道电压节数判定失败!") -> (w5441:string[])
                                n3895 = call "表格编辑.vi"("新元素/子数组"=w5441, "活动单元格:单元格背景色"=u32 16711680, "MCListbox引用句柄"=w5440) -> ()  [unwired: 9 out]
                                }
                                frame True {
                                }
                                }
                                }
                                frame 3 {
                                n3896 = case shown="假" w5442 {
                                frame False {
                                n3897 = control-ref of="结果"() -> (w5445:refnum<vi>)
                                n3898 = Build Array("保险位置判定失败!") -> (w5446:string[])
                                n3899 = call "表格编辑.vi"("新元素/子数组"=w5446, "活动单元格:单元格背景色"=u32 16711680, "MCListbox引用句柄"=w5445) -> ()  [unwired: 9 out]
                                }
                                frame True {
                                }
                                }
                                }
                                frame 4 {
                                n3900 = case shown="假" w5447 {
                                frame False {
                                n3901 = control-ref of="结果"() -> (w5450:refnum<vi>)
                                n3902 = Build Array("温度起始值判定失败!") -> (w5451:string[])
                                n3903 = call "表格编辑.vi"("新元素/子数组"=w5451, "活动单元格:单元格背景色"=u32 16711680, "MCListbox引用句柄"=w5450) -> ()  [unwired: 9 out]
                                }
                                frame True {
                                }
                                }
                                }
                                frame 5 {
                                n3904 = case shown="假" w5452 {
                                frame False {
                                n3905 = control-ref of="结果"() -> (w5455:refnum<vi>)
                                n3906 = Build Array("一级故障判定失败!") -> (w5456:string[])
                                n3907 = call "表格编辑.vi"("新元素/子数组"=w5456, "活动单元格:单元格背景色"=u32 16711680, "MCListbox引用句柄"=w5455) -> ()  [unwired: 9 out]
                                }
                                frame True {
                                }
                                }
                                }
                                frame 6 {
                                n3908 = case shown="假" w5457 {
                                frame False {
                                n3909 = control-ref of="结果"() -> (w5460:refnum<vi>)
                                n3910 = Build Array("二级故障判定失败!") -> (w5461:string[])
                                n3911 = call "表格编辑.vi"("新元素/子数组"=w5461, "活动单元格:单元格背景色"=u32 16711680, "MCListbox引用句柄"=w5460) -> ()  [unwired: 9 out]
                                }
                                frame True {
                                }
                                }
                                }
                                frame 7 {
                                n3912 = case shown="假" w5462 {
                                frame False {
                                n3913 = control-ref of="结果"() -> (w5465:refnum<vi>)
                                n3914 = Build Array("三级故障判定失败!") -> (w5466:string[])
                                n3915 = call "表格编辑.vi"("新元素/子数组"=w5466, "活动单元格:单元格背景色"=u32 16711680, "MCListbox引用句柄"=w5465) -> ()  [unwired: 9 out]
                                }
                                frame True {
                                }
